vi "sandbox.vi"() -> ()   [LabVIEW 2020]
uses:
  dt_encodeDecode.lvlib
panel:
  out "2s complement conversion ok":bool
  out "bcd conversion ok":bool
  out "decimal out":i16
  in  "size in bit":u8=9
  in  "decimal in":dbl
  out "decimal data out":u32
  out "bcd data out":u16 format="%016b"
  in  "size in bits":u32
  in  "word raw data - bcd":u16 format="%016b"
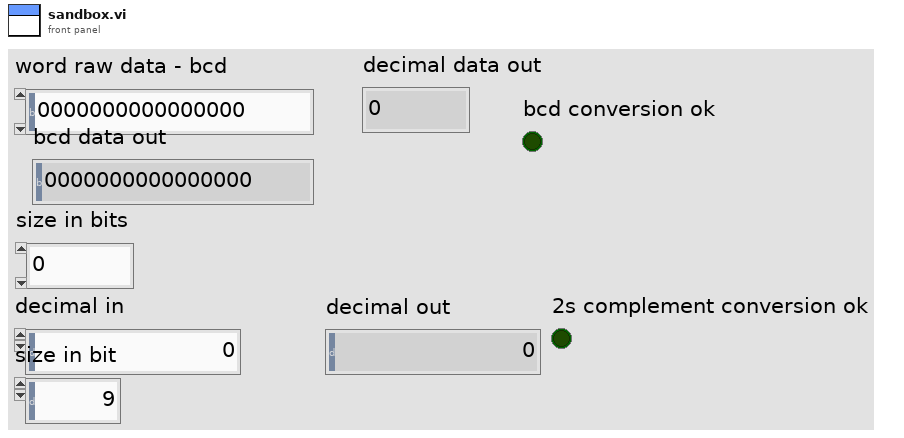
[diagram p1: front panel]
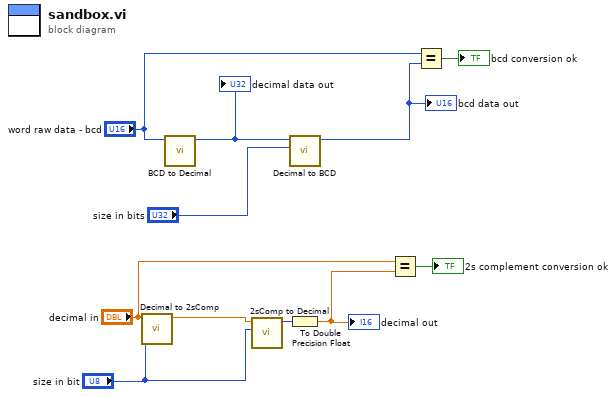
[diagram p0: block diagram]
diagram:
  n1 = call "Decimal to 2sComp.vi"("size in bit"="size in bit", "decimal in"="decimal in") -> ("word out"=w8:dbl)  [unwired: 9 in]
  n2 = call "BCD to Decimal.vi"("word raw data - bcd"="word raw data - bcd") -> ("decimal data out"=w11:u32)  [unwired: 10 in]
  "decimal data out" <- w11
  n3 = call "2sComp to Decimal.vi"("size in bit"="size in bit", "word in"=w8) -> ("decimal out"=w3:i16)  [unwired: 9 in]
  n4 = call "Decimal to BCD.vi"("size in bits"="size in bits", "decimal data in"=w11) -> ("bcd data out"=w6:u16)  [unwired: 9 in]
  "bcd data out" <- w6
  n5 = To Double Precision Float(number=w3) -> (double precision float=w1:dbl)
  "decimal out" <- w1
  n6 = Equal?(x="decimal in", y=w1) -> (x = y?=→"2s complement conversion ok":bool)
  n7 = Equal?(x="word raw data - bcd", y=w6) -> (x = y?=→"bcd conversion ok":bool)
